vi "Get Splitter Style (Core).vi"(6 "error in (no error)":errorcluster, 9 "Splitter in":refnum<vi>) -> (0 "error out":errorcluster, 3 "Style":T1 items=["Modern", "Classic", "System", "NXG"])   [LabVIEW 2015, in "Splitter.lvclass"]
uses:
  Splitter.lvclass
  Typedefs/Splitter Style--Enum.ctl
  Low-Level VI Manipulation/Find Resource by Type (String).vi
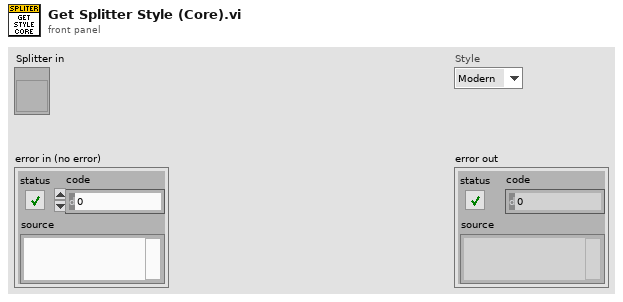
[diagram p1: front panel]
types:
  T1 = typedef "Splitter Style--Enum.ctl" = u16
  T2 = typedef "Resource Array.ctl" = T3[]
  T3 = typedef "Resource.ctl" = cluster{"type":u32, "id":i32, "name":string, "binary data":string}
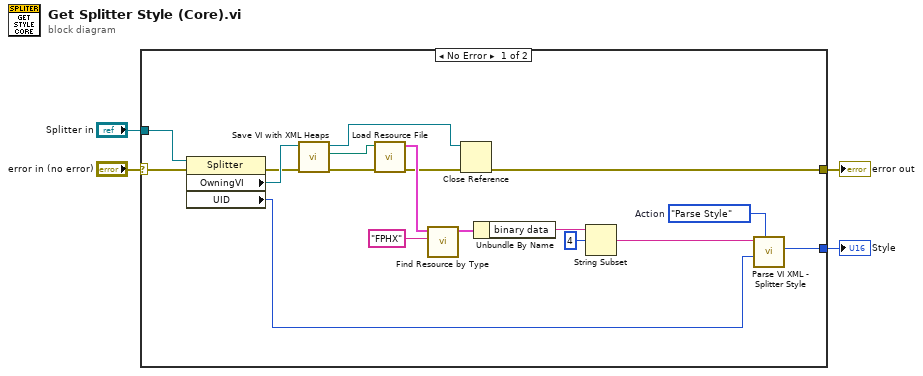
[diagram p0: block diagram]
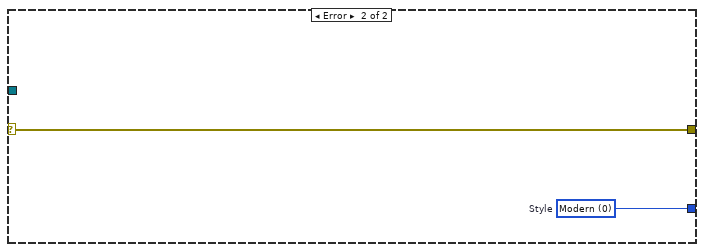
[diagram p2: hidden frame]
diagram:
  n1 = case shown="No Error" "error in (no error)" {
    selector: "error in (no error)" -> [w21 w24]
    tunnel: "Splitter in" -> [w22 _]
    tunnel: [w20 w24] -> w2
    tunnel: [w19 w23] -> w1
    frame No Error {
      w16 = enum16{"Parse Style", "Update Style"}."Parse Style"  # Action
      n2 = property class="Splitter"(reference=w22, error in=w21) -> (error out=w5:errorcluster, "OwningVI"=w6:refnum<vi>, "UID"=w18:i32)  [unwired: 1 out]
      n3 = call "Save VI with XML Heaps.vi"("error in (no error)"=w5, "VI Refnum In"=w6) -> ("error out"=w15:errorcluster, "VI Path out"=w9:path, "VI Refnum Out"=w7:refnum<vi>)  [unwired: 7 in]
      n4 = call "Load Resource File.vi"("error in (no error)"=w15, "Resource file"=w9) -> ("error out"=w8:errorcluster, "Resources"=w13:T2)  [unwired: 7 in, 1 out]
      n5 = call-poly "Find Resource by Type.vi"("Resource Type"="FPHX", "Resources"=w13) -> ("Resource"=w12:T3)  [unwired: 7 in, 2 out]
      n6 = Close Reference(reference=w7, error in (no error)=w8) -> (error out=w20:errorcluster)
      n7 = Unbundle By Name(w12) -> ("binary data"=w11:string)
      n8 = String Subset(string=w11, offset (0)=4) -> (substring=w17:string)  [unwired: 1 in]
      n9 = call "Parse VI XML - Splitter Style.vi"("Action"=w16, "UID"=w18, "VI XML in"=w17) -> ("Old Style"=w19:T1)  [unwired: 5 in, 1 out]
    }
    frame Error {
      w23 = T1 0 items=["Modern", "Classic", "System", "NXG"]  # Style
    }
  }
  "Style" <- w1
  "error out" <- w2
